vi "Write Single Register.vi"(8 "error in":errorcluster, 9 "register value":u16, 10 "address":u16, 11 "device data model in":refnum<class "Standard Data Model.lvclass">) -> (0 "error out":errorcluster, 3 "device data model out":refnum<class "Standard Data Model.lvclass">)   [LabVIEW 2013, in "Modbus Library - Advance.lvlib" / "Standard Data Model.lvclass"]
doc: "Writes the value of a single holding register."
uses:
  Standard Data Model.lvclass
  Standard Data Model.lvclass/Standard Data Model.ctl
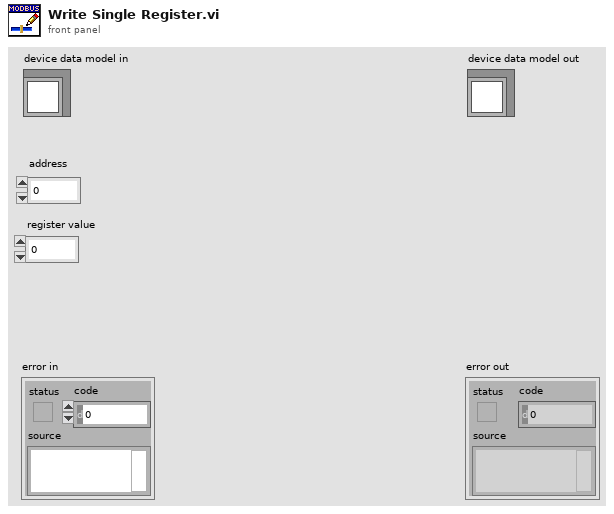
[diagram p1: front panel]
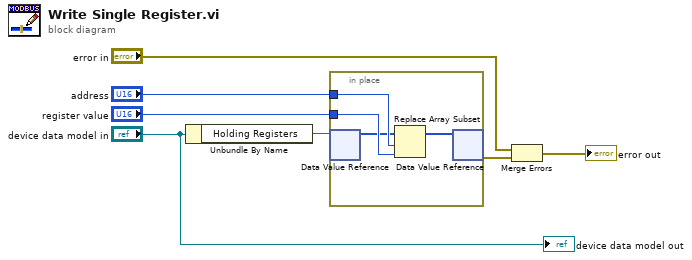
[diagram p0: block diagram]
diagram:
  n1 = Unbundle By Name("device data model in") -> ("Holding Registers"=w4:refnum<data-value>)
  n2 = in-place {
    in-place-border: "address" -> [w11]
    in-place-border: "register value" -> [w10]
    n3 = in-place-dvr #1(w4) -> (w9:u16[])  [unwired: 1 out]
    n4 = Replace Array Subset(array=w9, new element=w10, index=w11) -> (w8:u16[])
    n5 = in-place-dvr #1(w8) -> (w1:errorcluster)  [unwired: 1 out]
  }
  n6 = Merge Errors("error in", w1) -> (→"error out":errorcluster)
  "device data model out" <- "device data model in"
